vi "Clicked_Checkboxes.vi"(3 "Element Values in":enum8{"False", "True", "Mixed"}[](array[ring]), 4 "ElementFired":enum16{"Dialog", "PV", "Asynch", "Ack"}(ring)) -> (1 "Element Values out":enum8{"False", "True", "Mixed"}[](array[ring]), 5 "Element Status out Conditions":T1(array[ring]))   [LabVIEW 2016, in "CS++MessageMakerMain.lvlib" / "CS++MessageMakerMain.lvclass"]
uses:
  CS++MessageMakerMain.lvclass
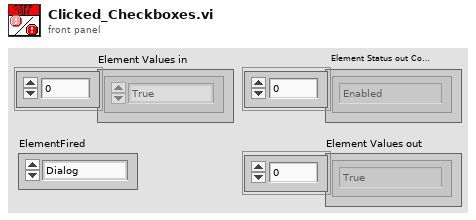
[diagram p1: front panel]
types:
  T1 = enum8{"Enabled", "Disabled", "Disabled and Grayed Out"}[]
  T2 = enum8{"Enabled", "Disabled", "Disabled and Grayed Out"}
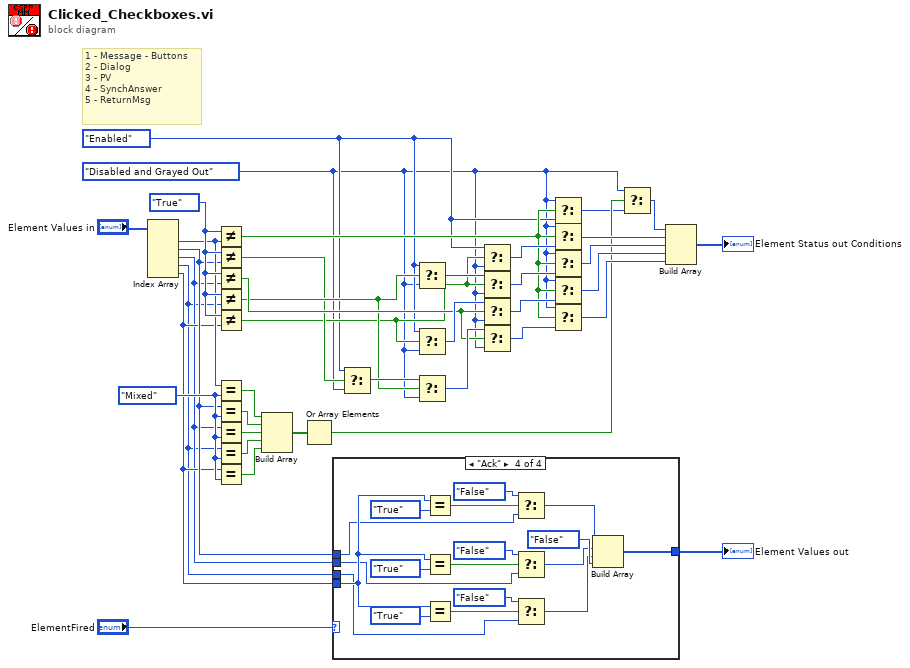
[diagram p0: block diagram]
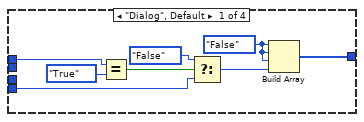
[diagram p2: hidden frame]
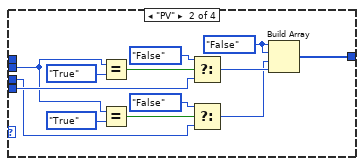
[diagram p3: hidden frame]
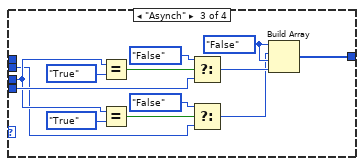
[diagram p4: hidden frame]
diagram:
  w17 = enum8{"False", "True", "Mixed"}."Mixed" ("y")
  w32 = enum8{"False", "True", "Mixed"}."True" ("y")
  w19 = T2."Enabled" ("Disabled")
  w8 = T2."Disabled and Grayed Out" ("t")
  # "1 - Message - Buttons\n2 - Dialog\n3 - PV\n4 - SynchAnswer\n5 - ReturnMsg"
  n1 = Index Array(array="Element Values in") -> (element #1=w18:enum8{"False", "True", "Mixed"}, element #2=w6:enum8{"False", "True", "Mixed"}, element #3=w2:enum8{"False", "True", "Mixed"}, element #4=w1:enum8{"False", "True", "Mixed"}, element #5=w5:enum8{"False", "True", "Mixed"})  [unwired: 5 in]
  n2 = Not Equal?(x=w32, y=w18) -> (x != y?=w20:bool)
  n3 = Not Equal?(x=w32, y=w6) -> (x != y?=w22:bool)
  n4 = Not Equal?(x=w32, y=w2) -> (x != y?=w24:bool)
  n5 = Not Equal?(x=w32, y=w1) -> (x != y?=w23:bool)
  n6 = Not Equal?(x=w32, y=w5) -> (x != y?=w21:bool)
  n7 = Equal?(x=w18, y=w17) -> (x = y?=w16:bool)
  n8 = Equal?(x=w6, y=w17) -> (x = y?=w15:bool)
  n9 = Equal?(x=w2, y=w17) -> (x = y?=w14:bool)
  n10 = Equal?(x=w1, y=w17) -> (x = y?=w13:bool)
  n11 = Equal?(x=w5, y=w17) -> (x = y?=w12:bool)
  n12 = Build Array(w16, w15, w14, w13, w12) -> (w11:bool[])
  n13 = Or Array Elements(Boolean array=w11) -> (logical OR=w9:bool)
  n14 = case shown="\"Ack\"" "ElementFired" {
    tunnel: w6 -> [w44 _ _ w76]
    tunnel: w5 -> [w43 w57 w70 w81]
    tunnel: [w40 w56 w69 w88] -> w4
    tunnel: w2 -> [_ w48 w61 w75]
    tunnel: w1 -> [_ w49 w62 w74]
    frame "Dialog", Default {
      w42 = enum8{"False", "True", "Mixed"}."False" ("Element Value")
      n15 = Equal?(x=w44, y=enum8{"False", "True", "Mixed"}."True") -> (x = y?=w47:bool)
      n16 = Select(t=enum8{"False", "True", "Mixed"}."False" ("Build AckReturn?"), s=w47, f=w43) -> (s? t:f=w41:enum8{"False", "True", "Mixed"})
      n17 = Build Array(w42, w42, w42, w41) -> (w40:enum8{"False", "True", "Mixed"}[])
    }
    frame "PV" {
      w54 = enum8{"False", "True", "Mixed"}."False" ("Element Value")
      n18 = Equal?(x=w48, y=enum8{"False", "True", "Mixed"}."True") -> (x = y?=w60:bool)
      n19 = Equal?(x=w48, y=enum8{"False", "True", "Mixed"}."True") -> (x = y?=w52:bool)
      n20 = Select(t=enum8{"False", "True", "Mixed"}."False" ("Build AckReturn?"), s=w60, f=w57) -> (s? t:f=w55:enum8{"False", "True", "Mixed"})
      n21 = Select(t=enum8{"False", "True", "Mixed"}."False" ("Build AckReturn?"), s=w52, f=w49) -> (s? t:f=w50:enum8{"False", "True", "Mixed"})
      n22 = Build Array(w54, w54, w50, w55) -> (w56:enum8{"False", "True", "Mixed"}[])
    }
    frame "Asynch" {
      w64 = enum8{"False", "True", "Mixed"}."False" ("Element Value")
      n23 = Equal?(x=w62, y=enum8{"False", "True", "Mixed"}."True") -> (x = y?=w73:bool)
      n24 = Equal?(x=w62, y=enum8{"False", "True", "Mixed"}."True") -> (x = y?=w66:bool)
      n25 = Select(t=enum8{"False", "True", "Mixed"}."False" ("Build AckReturn?"), s=w73, f=w70) -> (s? t:f=w68:enum8{"False", "True", "Mixed"})
      n26 = Select(t=enum8{"False", "True", "Mixed"}."False" ("Build AckReturn?"), s=w66, f=w61) -> (s? t:f=w63:enum8{"False", "True", "Mixed"})
      n27 = Build Array(w64, w63, w64, w68) -> (w69:enum8{"False", "True", "Mixed"}[])
    }
    frame "Ack" {
      n28 = Equal?(x=w81, y=enum8{"False", "True", "Mixed"}."True") -> (x = y?=w82:bool)
      n29 = Equal?(x=w81, y=enum8{"False", "True", "Mixed"}."True") -> (x = y?=w91:bool)
      n30 = Equal?(x=w81, y=enum8{"False", "True", "Mixed"}."True") -> (x = y?=w86:bool)
      n31 = Select(t=enum8{"False", "True", "Mixed"}."False" ("Build AckReturn?"), s=w82, f=w76) -> (s? t:f=w77:enum8{"False", "True", "Mixed"})
      n32 = Select(t=enum8{"False", "True", "Mixed"}."False" ("Build AckReturn?"), s=w91, f=w75) -> (s? t:f=w78:enum8{"False", "True", "Mixed"})
      n33 = Select(t=enum8{"False", "True", "Mixed"}."False" ("Build AckReturn?"), s=w86, f=w74) -> (s? t:f=w79:enum8{"False", "True", "Mixed"})
      n34 = Build Array(w77, w78, w79, enum8{"False", "True", "Mixed"}."False" ("Element Value")) -> (w88:enum8{"False", "True", "Mixed"}[])
    }
  }
  "Element Values out" <- w4
  n35 = Select(t=w19, s=w22, f=w8) -> (s? t:f=w25:T2)
  n36 = Select(t=w19, s=w23, f=w8) -> (s? t:f=w30:T2)
  n37 = Select(t=w19, s=w21, f=w8) -> (s? t:f=w27:T2)
  n38 = Select(t=w25, s=w23, f=w8) -> (s? t:f=w26:T2)
  n39 = Select(t=w19, s=w21, f=w8) -> (s? t:f=w33:T2)
  n40 = Select(t=w30, s=w21, f=w8) -> (s? t:f=w31:T2)
  n41 = Select(t=w27, s=w24, f=w8) -> (s? t:f=w29:T2)
  n42 = Select(t=w26, s=w24, f=w8) -> (s? t:f=w28:T2)
  n43 = Select(t=w8, s=w20, f=w19) -> (s? t:f=w7:T2)
  n44 = Select(t=w8, s=w20, f=w33) -> (s? t:f=w37:T2)
  n45 = Select(t=w8, s=w20, f=w31) -> (s? t:f=w36:T2)
  n46 = Select(t=w8, s=w20, f=w29) -> (s? t:f=w35:T2)
  n47 = Select(t=w8, s=w20, f=w28) -> (s? t:f=w34:T2)
  n48 = Select(t=w8, s=w9, f=w7) -> (s? t:f=w10:T2)
  n49 = Build Array(w10, w37, w36, w35, w34) -> (→"Element Status out Conditions":T1)
